vi "TCP - Ethernet Basic Communication.vi"(11 "Sync Packet":u8[](array[numeric])=[255, 7, 0, 0, 0, 0, 6]) -> (0 "Error Out":errorcluster={"status"=TRUE, "code"=62, "source"="TCP Write in TCP - Ethernet Basic Communication.vi"}, 3 "Return":u8[](array[numeric]))   [LabVIEW 2013]
uses:
  <vilib>/ptbypt/NI_PtbyPt.lvlib
panel:
  out "mean":dbl
  in  "Num Packets":i32=250
  in  "Read?":bool=TRUE
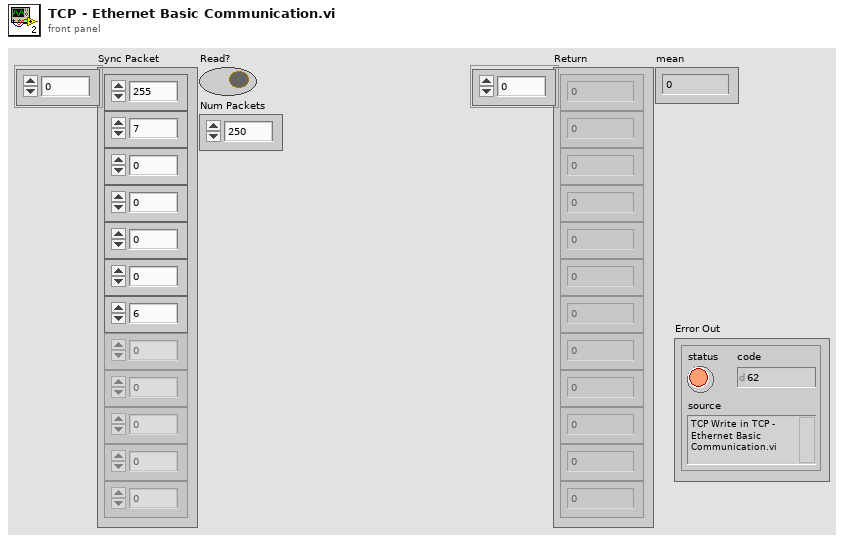
[diagram p1: front panel]
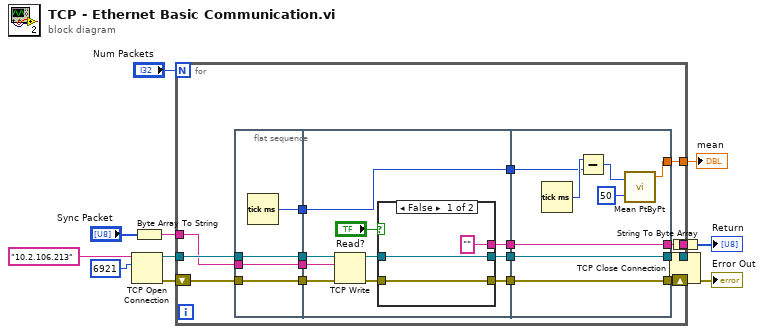
[diagram p0: block diagram]
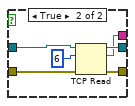
[diagram p2: hidden frame]
diagram:
  n1 = TCP Open Connection(address="10.2.106.213", remote port or service name=u16 6921) -> (connection ID=w13:refnum<k5>, error out=w12:errorcluster)  [unwired: 3 in]
  n2 = Byte Array To String(unsigned byte array="Sync Packet") -> (string=w9:string)
  n3 = for {
    N: "Num Packets" -> [_]
    tunnel: w13 -> [w28]
    tunnel: w9 -> [w26]
    tunnel: [w25] -> w6
    tunnel: [w23] -> w4
    shift-right: [w24] -> w5
    shift-left: w12 -> [w27]
    tunnel: [w14] -> w1
    n4 = flat-sequence {
      tunnel: w26 -> [w30]
      tunnel: w27 -> [w31]
      tunnel: w28 -> [w32]
      tunnel: [w32] -> w19
      tunnel: [w31] -> w18
      tunnel: [w30] -> w17
      tunnel: [w29] -> w16
      tunnel: [w38] -> w22
      tunnel: [w36] -> w21
      tunnel: [w35] -> w20
      tunnel: w19 -> [w42]
      tunnel: w18 -> [w41]
      tunnel: w17 -> [w40]
      tunnel: w16 -> [w33]
      tunnel: [w33] -> w15
      tunnel: [w57] -> w23
      tunnel: [w58] -> w24
      tunnel: [w59] -> w25
      tunnel: w22 -> [w59]
      tunnel: w21 -> [w58]
      tunnel: w20 -> [w57]
      tunnel: w15 -> [w55]
      tunnel: [w53] -> w14
      frame #0 {
        n5 = Tick Count (ms)() -> (millisecond timer value=w29:u32)
      }
      frame #1 {
        n6 = TCP Write(connection ID=w42, data in=w40, error in (no error)=w41) -> (connection ID out=w39:refnum<k5>, error out=w37:errorcluster)  [unwired: 1 in, 1 out]
        n7 = case shown="False" "Read?" {
          tunnel: w39 -> [w45 w51]
          tunnel: [w45 w50] -> w38
          tunnel: w37 -> [w44 w48]
          tunnel: [w44 w47] -> w36
          tunnel: ["" ("data out") w46] -> w35
          frame False {
          }
          frame True {
            n8 = TCP Read(connection ID=w51, bytes to read=6, error in (no error)=w48) -> (connection ID out=w50:refnum<k5>, data out=w46:string, error out=w47:errorcluster)  [unwired: 2 in]
          }
        }
      }
      frame #2 {
        n9 = Tick Count (ms)() -> (millisecond timer value=w56:u32)
        n10 = Subtract(x=w56, y=w55) -> (x-y=w52:u32)
        n11 = call <vilib>:"Mean PtByPt.vi"("x"=w52, "sample length"=50) -> ("mean"=w53:dbl)  [unwired: 2 in, 1 out]
      }
    }
  }
  "mean" <- w1
  n12 = String To Byte Array(string=w4) -> (unsigned byte array=→"Return":u8[])
  n13 = TCP Close Connection(connection ID=w6, error in (no error)=w5) -> (error out=→"Error Out":errorcluster)  [unwired: 1 in, 1 out]
